vi "Set2D_Magneticfield(polar)_PK.vi"(6 "Y-axis Ramp Rate (T/min)":string="0.004", 7 "Z-axis Ramp Rate (T/min)":string="0.004", 8 "Set target vector angle (degrees)":dbl=89.205 format="%#_13g", 9 "Set target vector magnitude (T)":dbl=2.2 format="%#_13g", 10 "Y-Axis Magnet IP Address":string="169.254.109.232", 11 "Z-Axis Magnet IP Address":string="169.254.239.127") -> (0 "Z-axis Magnetic Field (T)":string="2.199789387\r\n", 1 "Y-axis Magnetic Field (T)":string="0.030531683\r\n", 2 "q - Vector angle":dbl=89.20482193805654 format="%#_13g", 3 "R - Vector field magnitude (T)":dbl=2.2000012570052427 format="%#_13g")   [LabVIEW 2016]
panel:
  in  "?":bool
  out "Z-axis":dbl(slide)=2.199789387 scale=0.0..3.0
  out "Y-Axis":dbl(slide)=0.030531683 scale=0.0..3.0
  out "Y-axis Target Field setpoint (T)":string="0.030525"
  out "Y-axis Ramp rate (T/min)":dbl=0.004 format="%#_13g"
  out "Z-axis Target Field setpoint (T)":string="2.199788"
  out "Z-axis Ramp rate (T/min)":dbl=0.004 format="%#_13g"
  # "AMI 430 Magnet Set 2D Vector Field\nfor Bluefors LD-400 - PK v1.0\nZ-Axis: In-plane (90 deg)\nY-axis: Out-of-plane (0 deg)"
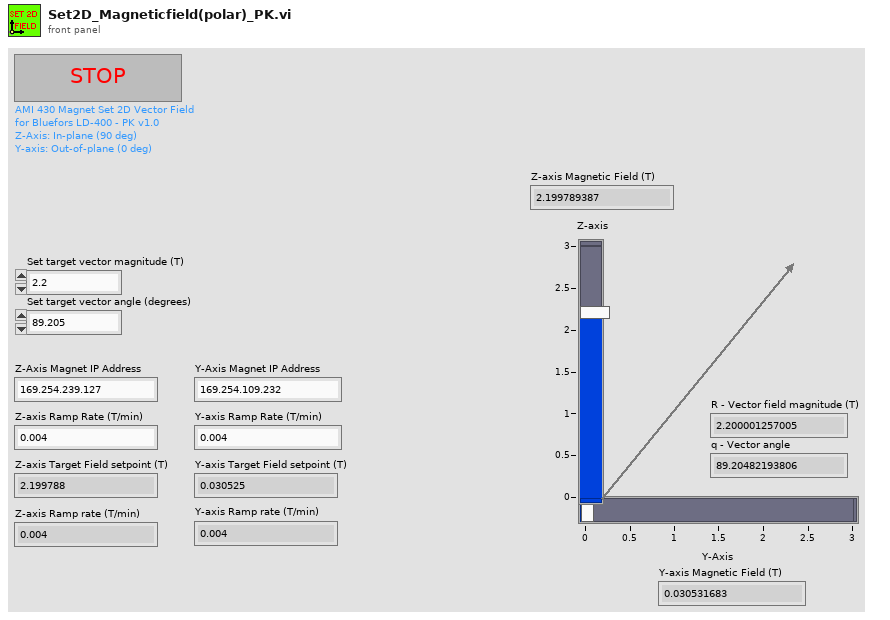
[diagram p1: front panel]
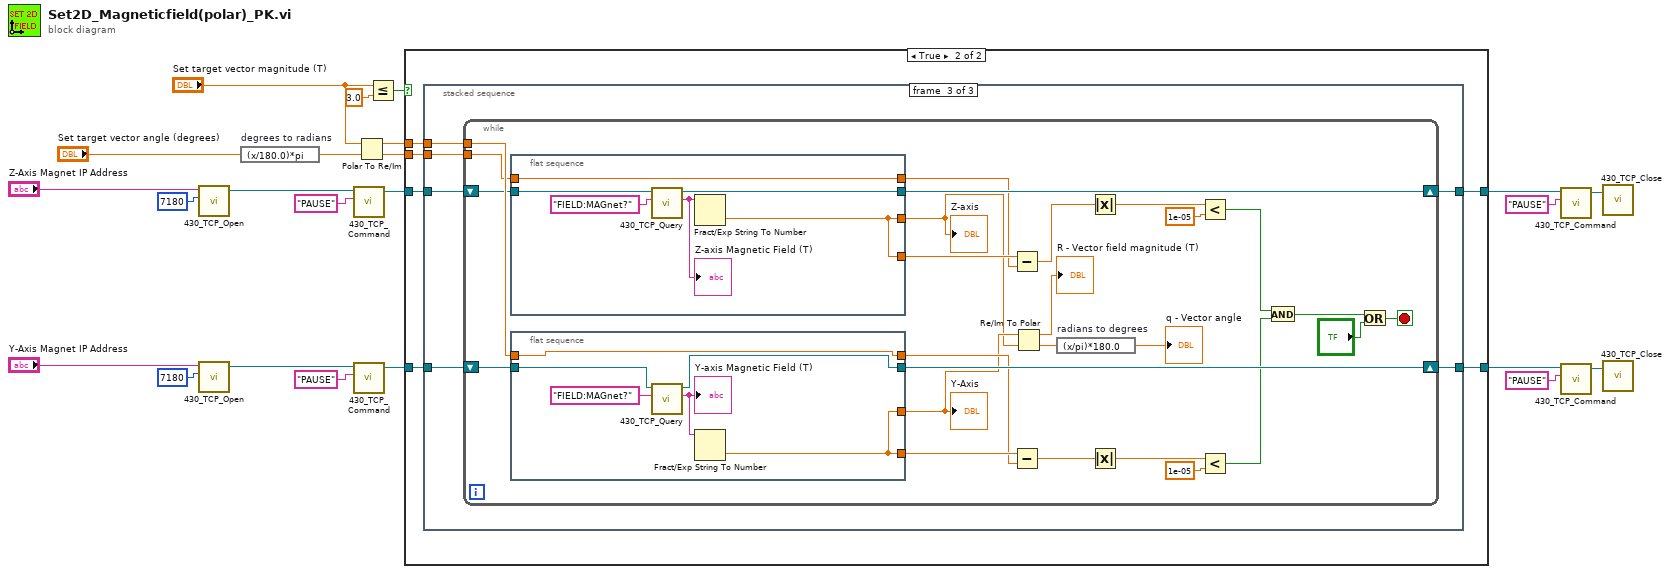
[diagram p0: block diagram]
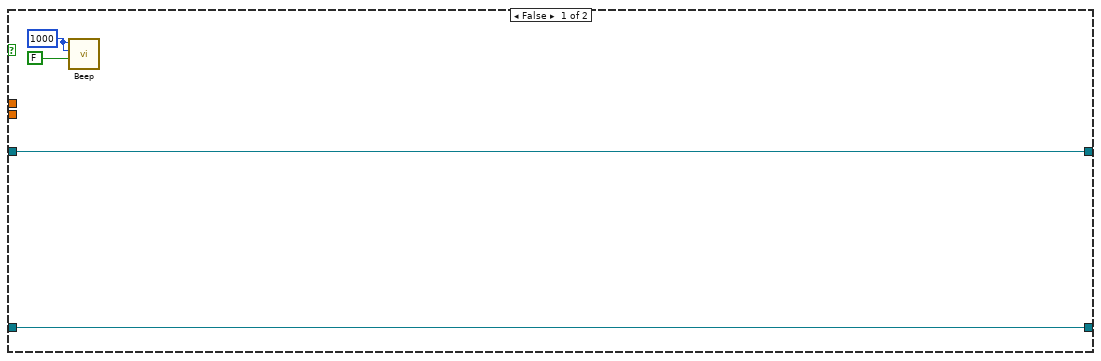
[diagram p2: hidden frame]
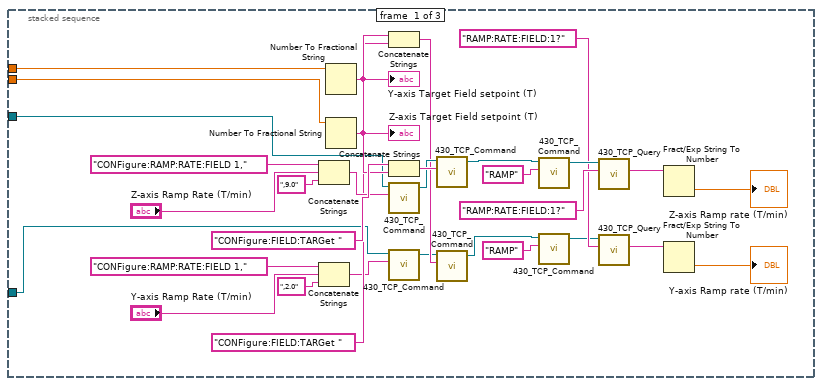
[diagram p3: hidden frame]
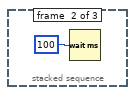
[diagram p4: hidden frame]
diagram:
  n1 = call "430_TCP_Open.vi"("IP Address"="Z-Axis Magnet IP Address", "TCP Port"=7180) -> ("connection ID"=w21:refnum<k5>)  [unwired: 4 in, 2 out]
  n2 = call "430_TCP_Open.vi"("IP Address"="Y-Axis Magnet IP Address", "TCP Port"=7180) -> ("connection ID"=w16:refnum<k5>)  [unwired: 4 in, 2 out]
  n3 = expression code="(x/180.0)*pi" "degrees to radians"("Set target vector angle (degrees)") -> (w10:dbl)
  n4 = call "430_TCP_Command.vi"("Command"="PAUSE", "connection ID"=w21) -> ("connection ID out"=w19:refnum<k5>)  [unwired: 2 in, 2 out]
  n5 = call "430_TCP_Command.vi"("Command"="PAUSE", "connection ID"=w16) -> ("connection ID out"=w14:refnum<k5>)  [unwired: 2 in, 2 out]
  n6 = Polar To Re/Im(2:w10, 3:"Set target vector magnitude (T)") -> (0:w7:dbl, 1:w8:dbl)
  n7 = Less Or Equal?(x="Set target vector magnitude (T)", y=3.0) -> (x <= y?=w12:bool)
  n8 = case shown="True" w12 {
    tunnel: w19 -> [w26 w32]
    tunnel: w14 -> [w27 w31]
    tunnel: [w26 w29] -> w3
    tunnel: [w27 w28] -> w2
    tunnel: w8 -> [_ w30]
    tunnel: w7 -> [_ w33]
    frame False {
      w24 = 1000
      n9 = call <vilib>:"Beep.vi"("use system alert? (T)"=FALSE, "duration (msec)"=w24, "frequency (Hz)"=w24) -> ()  [unwired: 9 in]
    }
    frame True {
      n10 = stacked-sequence {
        tunnel: w33 -> [w53 _ w69]
        tunnel: w32 -> [w50 _ w67]
        tunnel: w31 -> [w35 _ w68]
        tunnel: w30 -> [w34 _ w70]
        tunnel: [_ _ w72] -> w29
        tunnel: [_ _ w71] -> w28
        frame #0 {
          n11 = Concatenate Strings("CONFigure:RAMP:RATE:FIELD 1,", "Z-axis Ramp Rate (T/min)", ",9.0") -> (w54:string)
          n12 = Concatenate Strings("CONFigure:RAMP:RATE:FIELD 1,", "Y-axis Ramp Rate (T/min)", ",2.0") -> (w36:string)
          n13 = Number To Fractional String(number=w34) -> (F-format string=w40:string)  [unwired: 3 in]
          "Y-axis Target Field setpoint (T)" <- w40
          n14 = Number To Fractional String(number=w53) -> (F-format string=w58:string)  [unwired: 3 in]
          "Z-axis Target Field setpoint (T)" <- w58
          n15 = Concatenate Strings("CONFigure:FIELD:TARGet ", w40) -> (w42:string)
          n16 = Concatenate Strings("CONFigure:FIELD:TARGet ", w58) -> (w60:string)
          n17 = call "430_TCP_Command.vi"("Command"=w54, "connection ID"=w50) -> ("connection ID out"=w59:refnum<k5>)  [unwired: 2 in, 2 out]
          n18 = call "430_TCP_Command.vi"("Command"=w36, "connection ID"=w35) -> ("connection ID out"=w41:refnum<k5>)  [unwired: 2 in, 2 out]
          n19 = call "430_TCP_Command.vi"("Command"=w60, "connection ID"=w59) -> ("connection ID out"=w52:refnum<k5>)  [unwired: 2 in, 2 out]
          n20 = call "430_TCP_Command.vi"("Command"=w42, "connection ID"=w41) -> ("connection ID out"=w45:refnum<k5>)  [unwired: 2 in, 2 out]
          n21 = call "430_TCP_Command.vi"("Command"="RAMP", "connection ID"=w52) -> ("connection ID out"=w51:refnum<k5>)  [unwired: 2 in, 2 out]
          n22 = call "430_TCP_Command.vi"("Command"="RAMP", "connection ID"=w45) -> ("connection ID out"=w48:refnum<k5>)  [unwired: 2 in, 2 out]
          n23 = call "430_TCP_Query.vi"("Command"="RAMP:RATE:FIELD:1?" ("Magnetic Field (T)"), "connection ID"=w51) -> ("Response"=w63:string)  [unwired: 5 in, 4 out]
          n24 = call "430_TCP_Query.vi"("Command"="RAMP:RATE:FIELD:1?" ("Magnetic Field (T)"), "connection ID"=w48) -> ("Response"=w46:string)  [unwired: 5 in, 4 out]
          n25 = Fract/Exp String To Number(string=w63) -> (number=→"Z-axis Ramp rate (T/min)":dbl)  [unwired: 3 in, 1 out]
          n26 = Fract/Exp String To Number(string=w46) -> (number=→"Y-axis Ramp rate (T/min)":dbl)  [unwired: 3 in, 1 out]
        }
        frame #1 {
          n27 = Wait (ms)(milliseconds to wait=100) -> ()  [unwired: 1 out]
        }
        frame #2 {
          n28 = while {
            shift-right: [w97] -> w72
            shift-left: w67 -> [w82]
            shift-right: [w98] -> w71
            shift-left: w68 -> [w84]
            tunnel: w70 -> [w83]
            tunnel: w69 -> [w81]
            stop <- w80 stop-if-true
            n29 = flat-sequence {
              tunnel: [w103] -> w97
              tunnel: [w101] -> w96
              tunnel: [w99] -> w89
              tunnel: [w101] -> w73
              tunnel: w82 -> [w100]
              tunnel: w81 -> [w99]
              frame #0 {
                n30 = call "430_TCP_Query.vi"("Command"="FIELD:MAGnet?" ("Magnetic Field (T)"), "connection ID"=w100) -> ("Response"=w102:string, "connection ID out"=w103:refnum<k5>)  [unwired: 5 in, 3 out]
                "Z-axis Magnetic Field (T)" <- w102
                n31 = Fract/Exp String To Number(string=w102) -> (number=w101:dbl)  [unwired: 3 in, 1 out]
              }
            }
            n32 = flat-sequence {
              tunnel: [w109] -> w98
              tunnel: [w107] -> w91
              tunnel: [w105] -> w90
              tunnel: [w107] -> w74
              tunnel: w84 -> [w106]
              tunnel: w83 -> [w105]
              frame #0 {
                n33 = call "430_TCP_Query.vi"("Command"="FIELD:MAGnet?" ("Magnetic Field (T)"), "connection ID"=w106) -> ("Response"=w108:string, "connection ID out"=w109:refnum<k5>)  [unwired: 5 in, 3 out]
                "Y-axis Magnetic Field (T)" <- w108
                n34 = Fract/Exp String To Number(string=w108) -> (number=w107:dbl)  [unwired: 3 in, 1 out]
              }
            }
            n35 = Subtract(x=w96, y=w89) -> (x-y=w95:dbl)
            n36 = Subtract(x=w91, y=w90) -> (x-y=w93:dbl)
            n37 = Re/Im To Polar(2:w73, 3:w74) -> (0:w75:dbl, 1:→"R - Vector field magnitude (T)":dbl)
            n38 = expression code="(x/pi)*180.0" "radians to degrees"(w75) -> (→"q - Vector angle":dbl)
            n39 = Absolute Value(x=w95) -> (abs(x)=w94:dbl)
            n40 = Absolute Value(x=w93) -> (abs(x)=w92:dbl)
            n41 = Less?(x=w94, y=1e-05) -> (x < y?=w85:bool)
            n42 = Less?(x=w92, y=1e-05) -> (x < y?=w86:bool)
            n43 = And(x=w85, y=w86) -> (x .and. y?=w79:bool)
            n44 = Or(x=w79, y="?") -> (x .or. y?=w80:bool)
            "Z-axis" <- w73
            "Y-Axis" <- w74
          }
        }
      }
    }
  }
  n45 = call "430_TCP_Command.vi"("Command"="PAUSE", "connection ID"=w3) -> ("connection ID out"=w4:refnum<k5>)  [unwired: 2 in, 2 out]
  n46 = call "430_TCP_Command.vi"("Command"="PAUSE", "connection ID"=w2) -> ("connection ID out"=w1:refnum<k5>)  [unwired: 2 in, 2 out]
  n47 = call "430_TCP_Close.vi"("connection ID"=w4) -> ()  [unwired: 1 in, 2 out]
  n48 = call "430_TCP_Close.vi"("connection ID"=w1) -> ()  [unwired: 1 in, 2 out]
